vi "AUX_LineWrite.vi"(10 "String":string="#", 11 "Char Number":i32=40) -> (2 "Line Out":string)   [LabVIEW 2021]
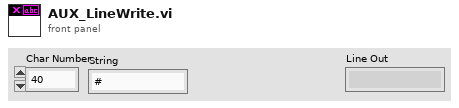
[diagram p1: front panel]
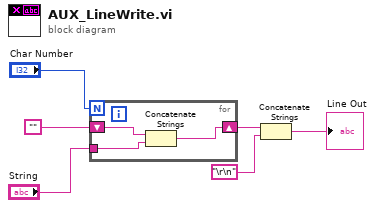
[diagram p0: block diagram]
diagram:
  n1 = for {
    N: "Char Number" -> [_]
    shift-right: [w8] -> w5
    shift-left: "" -> [w9]
    tunnel: "String" -> [w7]
    n2 = Concatenate Strings(w9, w7) -> (w8:string)
  }
  n3 = Concatenate Strings(w5, "\r\n") -> (→"Line Out":string)
